vi "State_ExecCMD.vi"(6 "Callback":T1, 8 "error in (no error)":errorcluster, 9 "Parameter":variant, 10 "Command":string, 11 "Formulas Module in":refnum<class "Formulas Module.lvclass">) -> (0 "error out":errorcluster, 1 "Suppress Debug?":bool, 2 "Debug Message":string, 3 "Formulas Module out":refnum<class "Formulas Module.lvclass">)   [LabVIEW 2021, in "Formulas Module.lvclass"]
uses:
  Formulas Module.lvclass
  C:/Program Files (x86)/National Instruments/LabVIEW 2021/user.lib/S2 Labs/Module Framework/Modules/Formulas/Formulas Base.lvclass
  C:/Program Files (x86)/National Instruments/LabVIEW 2021/user.lib/S2 Labs/Module Framework/Modules/Base/Module.lvclass
  <userlib>/S2 Labs/Module Framework/Modules/Base/Callback Typdef.ctl
  <userlib>/S2 Labs/Queued State Machine/Callback Notifier/Callback Notifier.lvclass
  <userlib>/S2 Labs/Queued State Machine/TypeDefs/CallbackNotifierRef.ctl
  <userlib>/S2 Labs/Module Framework/Modules/Formulas/Formulas Base.lvclass/Formulas Base.ctl
  <userlib>/S2 Labs/Queued State Machine/Callback Notifier/Callback Notifier.lvclass/Callback Notifier.ctl
  <userlib>/S2 Labs/Module Framework/Modules/Formulas/TypeDefs/Formula Config Element.ctl
  <userlib>/S2 Labs/Queued State Machine/TypeDefs/Queue Message.ctl
  <userlib>/S2 Labs/Queued State Machine/TypeDefs/States.ctl
  <userlib>/S2 Labs/Module Framework/Modules/Base/Module.lvclass/Module.ctl
  <userlib>/S2 Labs/Queued State Machine/QSM.lvclass/QSM.ctl
  b53aa1d4-834c-41fa-8069-a71bbcf985fc.vi
  <userlib>/S2 Labs/Module Framework/Modules/Formulas/Read Formulas Config.vi
  b773cab9-c153-489c-9824-3a9ce7061efa.vi
  79c68455-bbd7-483b-a53c-5bbade70d982.vi
  <userlib>/S2 Labs/Module Framework/Modules/Formulas/Write Initialized.vi
  <userlib>/S2 Labs/Module Framework/Modules/Formulas/Write Formulas Config.vi
  <userlib>/S2 Labs/Queued State Machine/Callback Notifier/Read Callback Notifier Ref.vi
  79c68455-bbd7-483b-a53c-5bbade70d982.vi/a5442550-30ab-4f7c-a4e8-4e040bcf3d57.vi
  <userlib>/S2 Labs/Module Framework/Modules/Base/Read Queue.vi
  79c68455-bbd7-483b-a53c-5bbade70d982.vi/77abbf80-a0d7-431e-91bd-d2268efe8bf3.vi
  79c68455-bbd7-483b-a53c-5bbade70d982.vi/7a27d807-84e4-485a-8ba6-289735576614.vi
  <userlib>/S2 Labs/Queued State Machine/Enqueue Element.vi
  <vilib>/Utility/error.llb/Error Cluster From Error Code.vi
  <userlib>/S2 Labs/Module Framework/Modules/Base/Get Module Queues Map.vi
  <userlib>/S2 Labs/Queued State Machine/Callback Notifier/Obtain Callback Notifier.vi
  <userlib>/S2 Labs/Queued State Machine/Callback Notifier/Release Reply Notifier.vi
  <vilib>/JDP Science/JSONtext/Variant to JSON Text.vi
  <userlib>/S2 Labs/Alarms and Events Toolkit/Alarms/Set User Event.vi
  <userlib>/S2 Labs/Queued State Machine/QSM.lvclass
  <vilib>/JDP Science/JSONtext/LVClass Serializer/JSONtext LVClass Serializer.lvclass
  <userlib>/S2 Labs/Module Framework/Modules/Formulas/Formulas Base.lvclass
  <userlib>/S2 Labs/Module Framework/Modules/Base/Module.lvclass
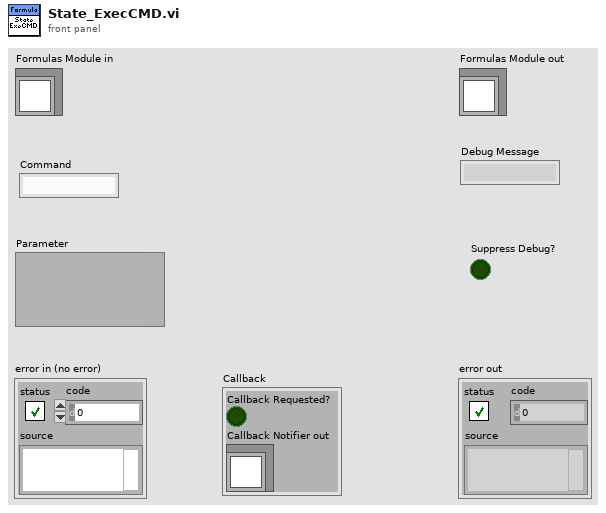
[diagram p1: front panel]
types:
  T1 = typedef "Module.lvclass/Callback Typdef.ctl" = cluster{"Callback Requested?":bool, "Callback Notifier out":T2}
  T2 = typedef "QSM.lvclass/CallbackNotifierRef.ctl" = refnum<class "Callback Notifier.lvclass">
  T3 = typedef "QSM.lvclass/Queue Message.ctl" = cluster{"State":T4, "Command":string, "Parameter":variant}
  T4 = typedef "QSM.lvclass/States.ctl" = enum16{"Waiting", "Init", "ExecCMD", "Read Config", "Write Config", "Launch", "Connect", "Recovery", "Clean Up", "Exit"}
  T5 = typedef "Formulas Base.lvclass/Formula Config Element.ctl" = cluster{"Name":string, "Formula":string, "Unit":string}
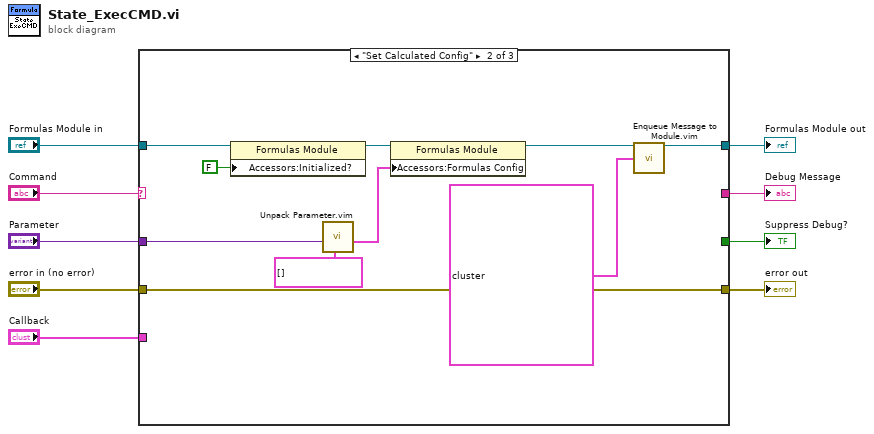
[diagram p0: block diagram]
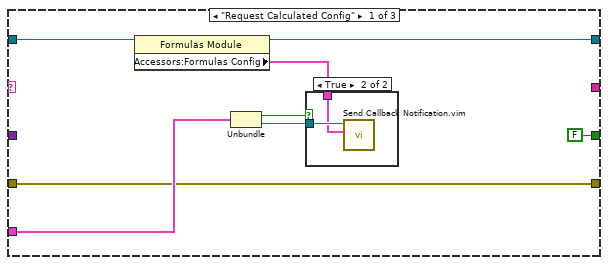
[diagram p2: hidden frame]
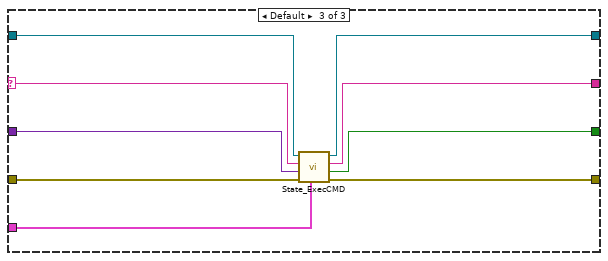
[diagram p4: hidden frame]
diagram:
  n1 = case shown="\"Set Calculated Config\"" "Command" {
    selector: "Command" -> [_ _ w31]
    tunnel: [w10 w21 w38] -> w9
    tunnel: [FALSE ("Suppress Debug?") _ w37] -> w8
    tunnel: [_ _ w36] -> w7
    tunnel: [w13 w22 w35] -> w6
    tunnel: "Callback" -> [w12 _ w34]
    tunnel: "error in (no error)" -> [w10 w21 w33]
    tunnel: "Parameter" -> [_ w20 w32]
    tunnel: "Formulas Module in" -> [w14 w23 w30]
    frame "Request Calculated Config" {
      n2 = property class="Formulas Module"(reference=w14) -> (reference out=w13:refnum<class "Formulas Module.lvclass">, "Accessors:Formulas Config"=w17:T5[])  [unwired: 1 in, 1 out]
      n3 = Unbundle(w12) -> ("Callback Requested?"=w16:bool, "Callback Notifier out"=w15:T2)
      n4 = case shown="True" w16 {
        tunnel: w15 -> [_ w19]
        tunnel: w17 -> [_ w18]
        frame False {
        }
        frame True {
          n5 = call "Send Callback Notification.vim"("notification (string)"=w18, "Callback Notifier in"=w19) -> ()  [unwired: 8 in, 2 out]
        }
      }
    }
    frame "Set Calculated Config" {
      n6 = property class="Formulas Module"(reference=w23, "Accessors:Initialized?"=FALSE ("_STATEVARS:Initialized?")) -> (reference out=w25:refnum<class "Formulas Module.lvclass">)  [unwired: 1 in, 1 out]
      n7 = call "Unpack Parameter.vim"("Parameter type (string)"=T5[] [] ("Array"), "Parameter Variant"=w20) -> ("Parameter"=w29:T5[])  [unwired: 8 in, 1 out]
      n8 = property class="Formulas Module"(reference=w25, "Accessors:Formulas Config"=w29) -> (reference out=w26:refnum<class "Formulas Module.lvclass">)  [unwired: 1 in, 1 out]
      n9 = call "Enqueue Message to Module.vim"("Module in"=w26, "Message"=T3[] [{"State"=enum."Write Config", "Command"="", "Parameter"=variant}, {"State"=enum."Init", "Command"="Unpack Formulas", "Parameter"=variant}, {"State"=enum."Init", "Command"="Init muParser", "Parameter"=variant}, {"State"=enum."Init", "Command"="Data Map", "Parameter"=variant}] ("Array")) -> ("Module out"=w22:refnum<class "Formulas Module.lvclass">)  [unwired: 8 in, 5 out]
    }
    frame Default {
      n10 = call-parent "State_ExecCMD.vi"("Callback"=w34, "error in (no error)"=w33, "Parameter"=w32, "Command"=w31, "Module in"=w30) -> ("error out"=w38:errorcluster, "Suppress Debug?"=w37:bool, "Debug Message"=w36:string, "Module out"=w35:refnum<class "Formulas Module.lvclass">)  [unwired: 3 in]
    }
  }
  "error out" <- w9
  "Formulas Module out" <- w6
  "Debug Message" <- w7
  "Suppress Debug?" <- w8
